vi "IMAQ FPGA Camera Link Counter.vi"(6 "Initializer Value":u32, 8 "Restart Value":u32, 9 "Restart?":bool, 10 "Increment Amount":u32=1, 11 "Increment?":bool) -> (3 "Count":u32)   [LabVIEW 2020]
doc: "This VI implements a configurable 32-bit counter. It has the ability to increment and restart when needed. The initial value and the restart value can be configured."
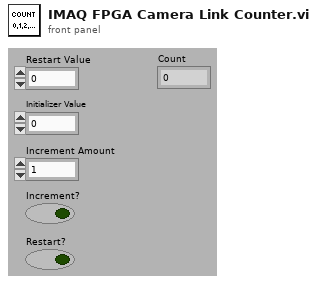
[diagram p1: front panel]
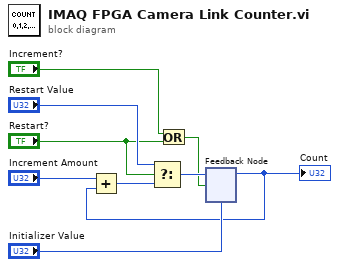
[diagram p0: block diagram]
diagram:
  n1 = Or(x="Increment?", y="Restart?") -> (x .or. y?=w1:bool)
  n2 = feedback #1("Initializer Value") -> (w6:u32)
  "Count" <- w6
  n3 = Add(x="Increment Amount", y=w6) -> (x+y=w5:u32)
  n4 = Select(t="Restart Value", s="Restart?", f=w5) -> (s? t:f=w4:u32)
  n5 = feedback-in #1(w4, w1) -> ()
